vi "LoadGlobais2.vi"(8 "error in (no error)":errorcluster, 10 "Mecanismo":string, 11 "QuickSilver in":refnum<class "QuickSilver.lvclass">) -> (0 "error out":errorcluster, 2 "Resp":string, 3 "QuickSilver out":refnum<class "QuickSilver.lvclass">)   [LabVIEW 2012, in "QuickSilver.lvclass"]
uses:
  QuickSilver.lvclass
  Global Coude.vi
  <vilib>/Utility/config.llb/NI_LVConfig.lvlib
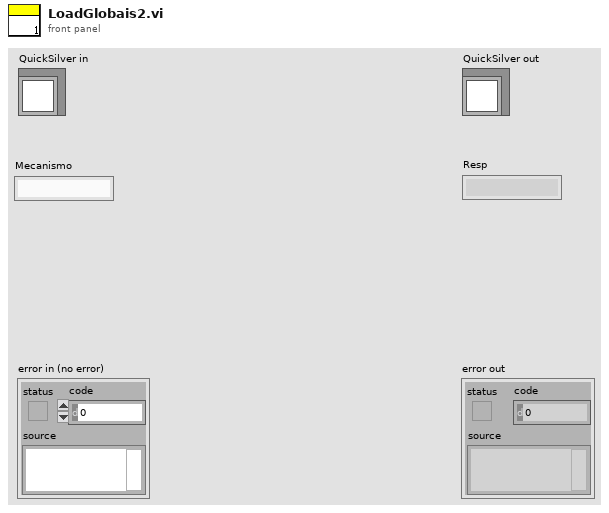
[diagram p1: front panel]
types:
  T1 = cluster{"Mec ID":string, "VISA Mec":refnum<visa-resource-name>, "Mec PosLimit":string, "Mec NegLimit":string, "Mec Factor":dbl, "Mec Speed":dbl, "Mec Acceleration":dbl, "MecOffset":string, "MecTargets":dbl[], "MecEnabled":bool, "Mec Target":dbl}
  T2 = typedef "NI_LVConfig.lvlib/Config Data RefNum.ctl" = refnum<k1>
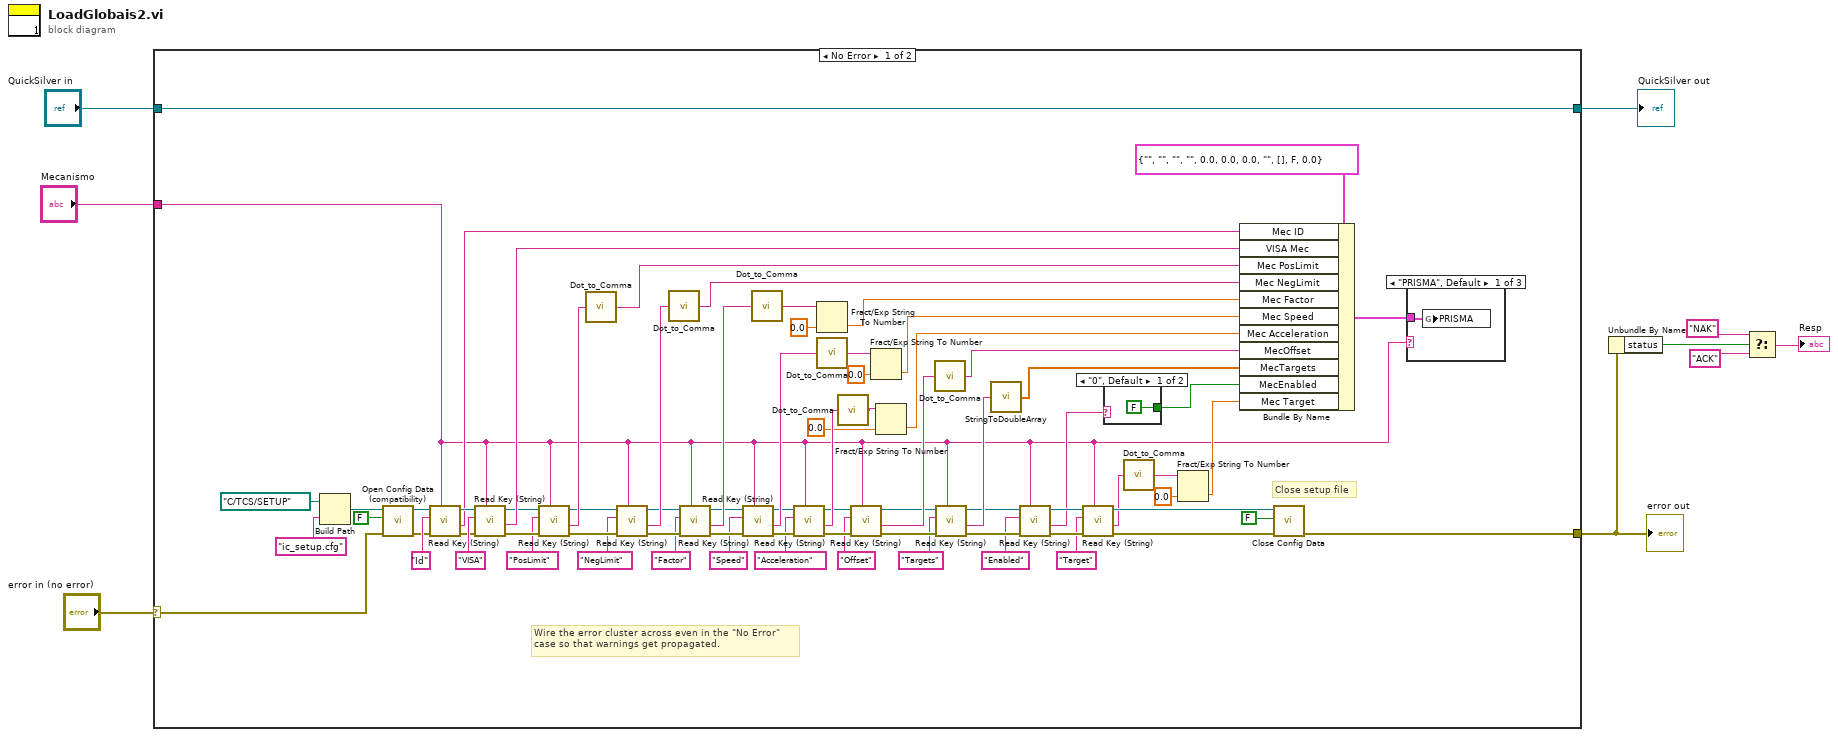
[diagram p0: block diagram]
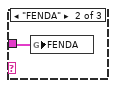
[diagram p2: hidden frame]
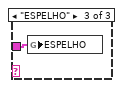
[diagram p3: hidden frame]
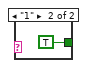
[diagram p4: hidden frame]
diagram:
  n1 = case shown="No Error" "error in (no error)" {
    selector: "error in (no error)" -> [w14 w90]
    tunnel: [w13 w90] -> w2
    tunnel: [w12 w89] -> w8
    tunnel: "QuickSilver in" -> [w12 w89]
    tunnel: "Mecanismo" -> [w10 _]
    frame No Error {
      # "Close setup file"
      # "Wire the error cluster across even in the \"No Error\"\ncase so that warnings get propagated."
      n2 = Build Path(base path=path "C:/TCS/SETUP", name or relative path="ic_setup.cfg") -> (appended path=w20:path)
      n3 = call <vilib>:"Open Config Data (compatibility).vi"("error in (no error)"=w14, "create file if necessary (T)"=FALSE ("create file if necessary? (T)"), "configuration file path"=w20) -> ("error out"=w18:errorcluster, "refnum"=w17:T2)  [unwired: 6 in, 1 out]
      n4 = call <vilib>:"Read Key (String).vi"("section"=w10, "error in (no error)"=w18, "key"="Id", "refnum"=w17) -> ("error out"=w22:errorcluster, "value"=w21:string, "refnum out"=w23:T2)  [unwired: 2 in, 3 out]
      n5 = call <vilib>:"Read Key (String).vi"("section"=w10, "error in (no error)"=w22, "key"="VISA", "refnum"=w23) -> ("error out"=w62:errorcluster, "value"=w76:string, "refnum out"=w58:T2)  [unwired: 2 in, 3 out]
      n6 = call <vilib>:"Read Key (String).vi"("section"=w10, "error in (no error)"=w62, "key"="PosLimit", "refnum"=w58) -> ("error out"=w64:errorcluster, "value"=w68:string, "refnum out"=w63:T2)  [unwired: 2 in, 3 out]
      n7 = call "Dot_to_Comma.vi"("String in"=w68) -> ("String out"=w77:string)
      n8 = call <vilib>:"Read Key (String).vi"("section"=w10, "error in (no error)"=w64, "key"="NegLimit", "refnum"=w63) -> ("error out"=w61:errorcluster, "value"=w69:string, "refnum out"=w57:T2)  [unwired: 2 in, 3 out]
      n9 = call "Dot_to_Comma.vi"("String in"=w69) -> ("String out"=w78:string)
      n10 = call <vilib>:"Read Key (String).vi"("section"=w10, "error in (no error)"=w61, "key"="Factor", "refnum"=w57) -> ("error out"=w60:errorcluster, "value"=w70:string, "refnum out"=w56:T2)  [unwired: 2 in, 3 out]
      n11 = call <vilib>:"Read Key (String).vi"("section"=w10, "error in (no error)"=w60, "key"="Speed", "refnum"=w56) -> ("error out"=w59:errorcluster, "value"=w66:string, "refnum out"=w55:T2)  [unwired: 2 in, 3 out]
      n12 = call "Dot_to_Comma.vi"("String in"=w70) -> ("String out"=w71:string)
      n13 = call <vilib>:"Read Key (String).vi"("section"=w10, "error in (no error)"=w59, "key"="Acceleration", "refnum"=w55) -> ("error out"=w50:errorcluster, "value"=w72:string, "refnum out"=w49:T2)  [unwired: 2 in, 3 out]
      n14 = Fract/Exp String To Number(string=w71, default (0 dbl)=0.0 ("default (0 DBL)")) -> (number=w79:dbl)  [unwired: 3 out]
      n15 = call "Dot_to_Comma.vi"("String in"=w66) -> ("String out"=w67:string)
      n16 = call "Dot_to_Comma.vi"("String in"=w72) -> ("String out"=w73:string)
      n17 = call <vilib>:"Read Key (String).vi"("section"=w10, "error in (no error)"=w50, "key"="Offset", "refnum"=w49) -> ("error out"=w48:errorcluster, "value"=w74:string, "refnum out"=w47:T2)  [unwired: 2 in, 3 out]
      n18 = Fract/Exp String To Number(string=w67, default (0 dbl)=0.0) -> (number=w80:dbl)  [unwired: 3 out]
      n19 = Fract/Exp String To Number(string=w73, default (0 dbl)=0.0) -> (number=w81:dbl)  [unwired: 3 out]
      n20 = call "Dot_to_Comma.vi"("String in"=w74) -> ("String out"=w82:string)
      n21 = call <vilib>:"Read Key (String).vi"("section"=w10, "error in (no error)"=w48, "key"="Targets", "refnum"=w47) -> ("error out"=w35:errorcluster, "value"=w40:string, "refnum out"=w38:T2)  [unwired: 2 in, 3 out]
      n22 = call "StringToDoubleArray.vi"("String"=w40) -> ("MecTargets"=w83:dbl[])
      n23 = call <vilib>:"Read Key (String).vi"("section"=w10, "error in (no error)"=w35, "key"="Enabled", "refnum"=w38) -> ("error out"=w34:errorcluster, "value"=w30:string, "refnum out"=w37:T2)  [unwired: 2 in, 3 out]
      n24 = call <vilib>:"Read Key (String).vi"("section"=w10, "error in (no error)"=w34, "key"="Target", "refnum"=w37) -> ("error out"=w33:errorcluster, "value"=w26:string, "refnum out"=w36:T2)  [unwired: 2 in, 3 out]
      n25 = case shown="\"0\", Default" w30 {
        tunnel: [FALSE TRUE] -> w29
        frame "0", Default {
        }
        frame "1" {
        }
      }
      n26 = call "Dot_to_Comma.vi"("String in"=w26) -> ("String out"=w28:string)
      n27 = Fract/Exp String To Number(string=w28, default (0 dbl)=0.0) -> (number=w25:dbl)  [unwired: 3 out]
      n28 = Bundle By Name(cluster=T1 {"Mec ID"="", "VISA Mec"="", "Mec PosLimit"="", "Mec NegLimit"="", "Mec Factor"=0.0, "Mec Speed"=0.0, "Mec Acceleration"=0.0, "MecOffset"="", "MecTargets"=[], "MecEnabled"=FALSE, "Mec Target"=0.0} ("CAM"), "Mec ID"=w21, "VISA Mec"=w76, "Mec PosLimit"=w77, "Mec NegLimit"=w78, "Mec Factor"=w79, "Mec Speed"=w80, "Mec Acceleration"=w81, "MecOffset"=w82, "MecTargets"=w83, "MecEnabled"=w29, "Mec Target"=w25) -> (w16:T1)
      n29 = call <vilib>:"Close Config Data.vi"("error in (no error)"=w33, "write file if changed (T)"=FALSE ("create file if necessary? (T)"), "refnum"=w36) -> ("error out"=w13:errorcluster)  [unwired: 8 out]
      n30 = case shown="\"PRISMA\", Default" w10 {
        tunnel: w16 -> [w84 w85 w86]
        frame "PRISMA", Default {
          n31 = global write "Global Coude.vi" "PRISMA"(w84) -> ()
        }
        frame "FENDA" {
          n32 = global write "Global Coude.vi" "FENDA"(w85) -> ()
        }
        frame "ESPELHO" {
          n33 = global write "Global Coude.vi" "ESPELHO"(w86) -> ()
        }
      }
    }
    frame Error {
    }
  }
  "error out" <- w2
  "QuickSilver out" <- w8
  n34 = Unbundle By Name(w2) -> ("status"=w6:bool)
  n35 = Select(t="NAK", s=w6, f="ACK") -> (s? t:f=→"Resp":string)
